vi "example test.vi"() -> ()   [LabVIEW 2013, in "scan engine tests.lvlib"]
uses:
  scan engine tests.lvlib
  <vilib>/NI/Tag Bus/table/allocation specification.ctl
  <vilib>/NI/Tag Bus/tag/Data Type.ctl
  <vilib>/NI/Tag Bus/dictionary/full data dictionary.ctl
  configuration/Scan Engine configuration.lvclass
  execution/Scan Engine runtime.lvclass
  <vilib>/NI/Tag Bus Module Framework/channel/channel classification.ctl
  configuration/Scan Engine configuration.lvclass/Scan Engine configuration.ctl
  <vilib>/NI/Tag Bus/table/data polymorphs/write one/write Boolean.vi
  <vilib>/NI/Tag Bus/table/data polymorphs/read one/read Double.vi
  configuration/Write discover channels.vi
  <vilib>/NI/Tag Bus/table/data table.lvlib
  <vilib>/NI/Tag Bus/dictionary/data dictionary.lvclass
  <vilib>/NI/Tag Bus Module Framework/channel/TBM channel.lvclass
  <vilib>/NI/Tag Bus/tag/tag descriptor.lvclass
panel:
  out "out":T1
  out "in":T1
  in  "do0 value":bool
  out "usec/run out":dbl
  out "usec/run in":dbl
  out "input count":T2[](array[typedef])
  out "output count":T2[](array[typedef])
  in  "for count":i32=1000
  out "AI0 value":dbl
  out "final error":errorcluster
  out "output error":errorcluster
  out "input error":errorcluster
  out "output lookup error":errorcluster
  out "input lookup error":errorcluster
  out "init error":errorcluster
  out "correct execution settings":bool
  out "serialization problem":errorcluster
  out "invalid configuration":errorcluster
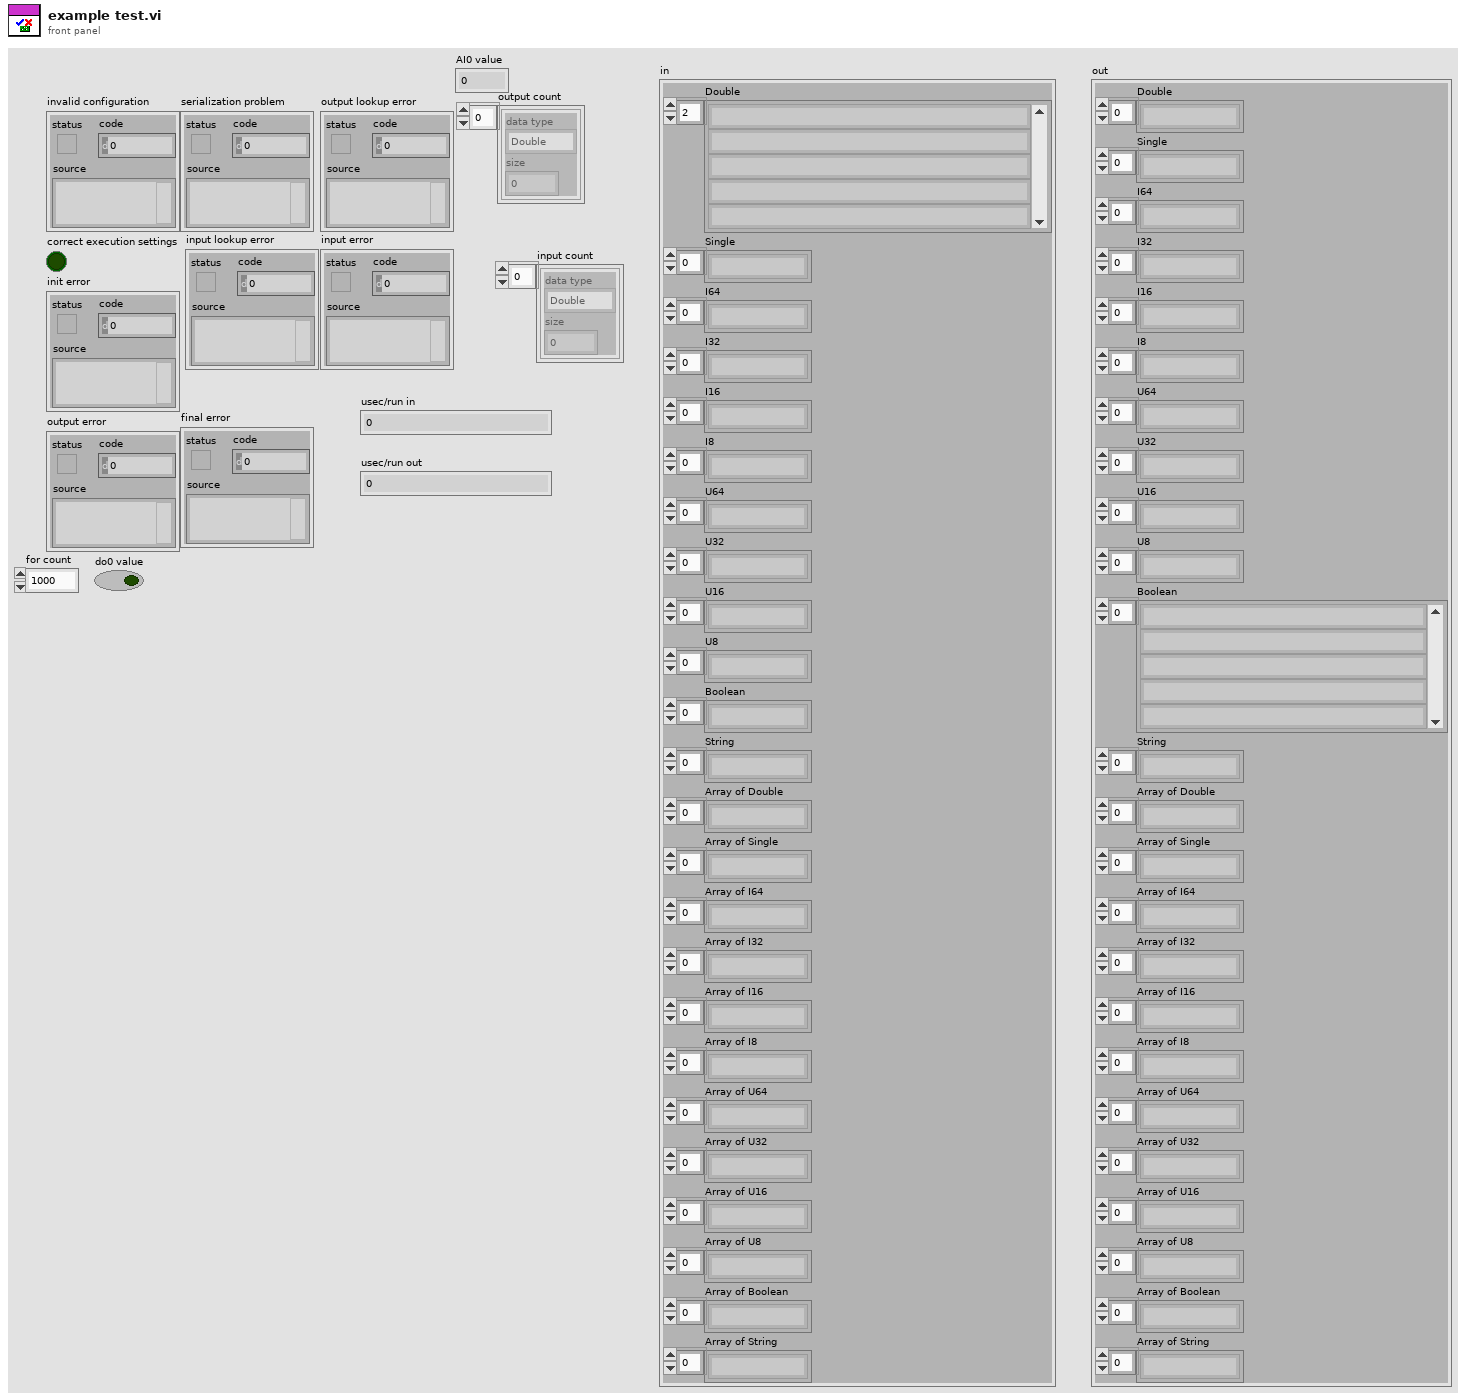
[diagram p1: front panel]
types:
  T1 = typedef "tag bus.lvlib/data dictionary.lvclass/full data dictionary.ctl" = cluster{"Double":string[], "Single":string[], "I64":string[], "I32":string[], "I16":string[], "I8":string[], "U64":string[], "U32":string[], "U16":string[], "U8":string[], "Boolean":string[], "String":string[], "Array of Double":string[], "Array of Single":string[], "Array of I64":string[], "Array of I32":string[], "Array of I16":string[], "Array of I8":string[], "Array of U64":string[], "Array of U32":string[], "Array of U16":string[], "Array of U8":string[], "Array of Boolean":string[], "Array of String":string[]}
  T2 = typedef "tag bus.lvlib/data table.lvlib/allocation specification.ctl" = cluster{"data type":T3, "size":i32}
  T3 = typedef "tag bus.lvlib/tag descriptor.lvclass/Data Type.ctl" = enum16{"Double", "Single", "I64", "I32", "I16", "I8", "U64", "U32", "U16", "U8", "Boolean", "String", "Array of Double", "Array of Single", "Array of I64", "Array of I32", "Array of I16", "Array of I8", "Array of U64", "Array of U32", "Array of U16", "Array of U8", "Array of Boolean", "Array of String"}
  T4 = typedef "TBM channel.lvclass/channel classification.ctl" = enum16{"input data", "output data", "processing parameter", "processing result"}
  T5 = typedef "TBM channel.lvclass/data tables.ctl" = cluster{"input data":T6, "processing parameter":T6, "processing result":T6, "output data":T6}
  T6 = typedef "tag bus.lvlib/dictionary table pair.ctl" = cluster{"data dictionary":refnum<class "data dictionary.lvclass">, "data table":T7}
  T7 = typedef "tag bus.lvlib/data table.lvlib/data table.ctl" = cluster{"Double":dbl[], "Single":sgl[], "I64":i64[], "I32":i32[], "I16":i16[], "I8":i8[], "U64":u64[], "U32":u32[], "U16":u16[], "U8":u8[], "Boolean":bool[], "String":string[], "Array of Double":cluster{"DBL Array":dbl[]}[], "Array of Single":cluster{"SGL Array":sgl[]}[], "Array of I64":cluster{"I64 Array":i64[]}[], "Array of I32":cluster{"I32 Array":i32[]}[], "Array of I16":cluster{"I16 Array":i16[]}[], "Array of I8":cluster{"I8 Array":i8[]}[], "Array of U64":cluster{"U64 Array":u64[]}[], "Array of U32":cluster{"U32 Array":u32[]}[], "Array of U16":cluster{"U16 Array":u16[]}[], "Array of U8":cluster{"U8 Array":u8[]}[], "Array of Boolean":cluster{"Boolean Array":bool[]}[], "Array of String":cluster{"String Array":string[]}[]}
  T8 = typedef "TBM module execution interface.lvclass/execution settings.ctl" = cluster{"reads inputs":bool, "processes data":bool, "writes outputs":bool}
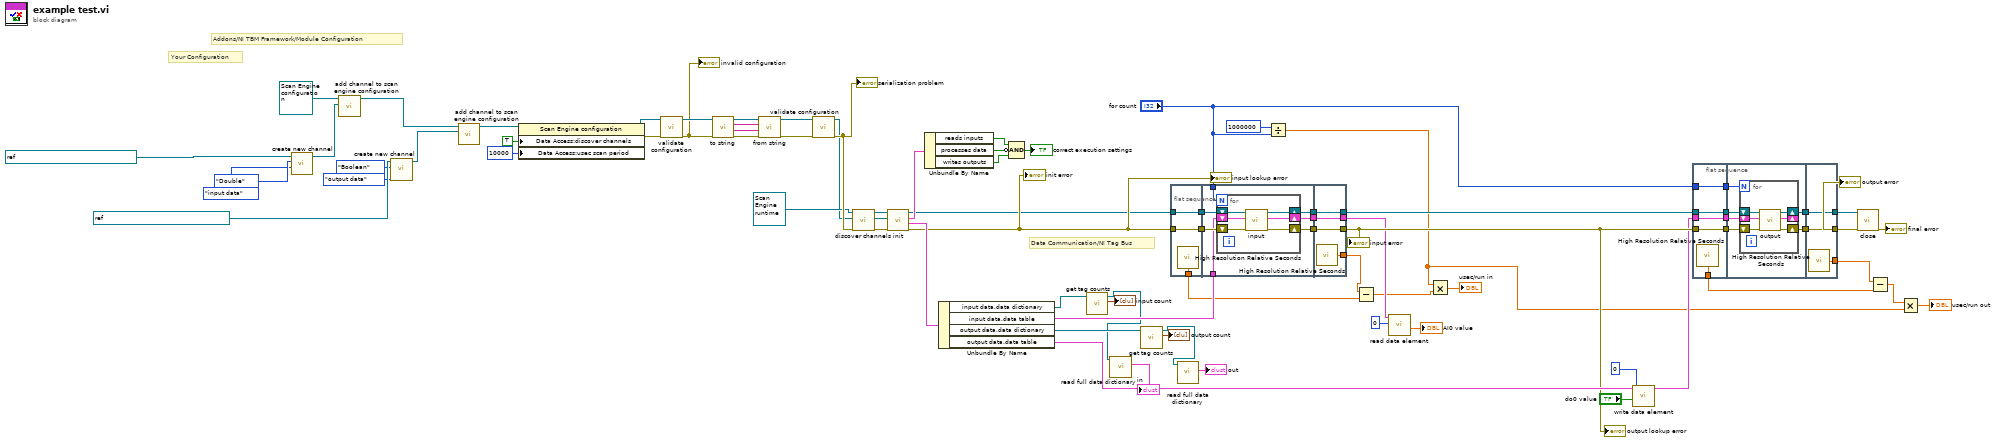
[diagram p0: block diagram]
diagram:
  # "Data Communication/NI Tag Bus"
  # "Your Configuration"
  # "Addons/NI TBM Framework/Module Configuration"
  n1 = call <vilib>:"create new channel.vi"("channel classification"=channel_classification."input data", "data type"=Data_Type."Double", "channel name"=refnum<k21> "ni.var.io://localhost/Mod1/AI0" ("shared variable refnum in")) -> ("channel"=w14:refnum<class "TBM channel.lvclass">)  [unwired: 8 in]
  n2 = call "add channel to scan engine configuration.vi"("channel"=w14, "Scan Engine configuration in"=refnum<class "Scan Engine configuration.lvclass"> refnum ("Scan Engine configuration")) -> ("Scan Engine configuration out"=w15:refnum<class "Scan Engine configuration.lvclass">)  [unwired: 8 in, 1 out]
  n3 = call <vilib>:"create new channel.vi"("channel classification"=channel_classification."output data", "data type"=Data_Type."Boolean", "channel name"=refnum<k21> "ni.var.io://localhost/Mod2/DO0" ("shared variable refnum in")) -> ("channel"=w13:refnum<class "TBM channel.lvclass">)  [unwired: 8 in]
  n4 = call "add channel to scan engine configuration.vi"("channel"=w13, "Scan Engine configuration in"=w15) -> ("Scan Engine configuration out"=w16:refnum<class "Scan Engine configuration.lvclass">)  [unwired: 8 in, 1 out]
  n5 = property class="Scan Engine configuration"(reference=w16, "Data Access:discover channels"=TRUE ("discover channels"), "Data Access:usec scan period"=u32 10000 ("scan period (uSec)")) -> (reference out=w56:refnum<class "Scan Engine configuration.lvclass">, error out=w55:errorcluster)  [unwired: 1 in]
  n6 = call-dynamic "validate configuration.vi"("error in"=w55, "Scan Engine configuration in"=w56) -> ("error out"=w79:errorcluster, "Scan Engine configuration out"=w80:refnum<class "Scan Engine configuration.lvclass">)  [unwired: 8 in]
  "invalid configuration" <- w79
  n7 = call-dynamic "to string.vi"("error in"=w79, "Scan Engine configuration in"=w80) -> ("error out"=w75:errorcluster, "data"=w76:string, "version"=w77:string, "Scan Engine configuration out"=w78:refnum<class "Scan Engine configuration.lvclass">)  [unwired: 6 in]
  n8 = call-dynamic "from string.vi"("error in"=w75, "data"=w76, "version"=w77, "Scan Engine configuration in"=w78) -> ("error out"=w73:errorcluster, "Scan Engine configuration out"=w74:refnum<class "Scan Engine configuration.lvclass">)  [unwired: 6 in]
  n9 = call-dynamic "validate configuration.vi"("error in"=w73, "Scan Engine configuration in"=w74) -> ("error out"=w51:errorcluster, "Scan Engine configuration out"=w46:refnum<class "Scan Engine configuration.lvclass">)  [unwired: 8 in]
  "serialization problem" <- w51
  n10 = call-dynamic "discover channels.vi"("error in"=w51, "module configuration"=w46, "module in"=refnum<class "Scan Engine runtime.lvclass"> refnum ("Scan Engine runtime")) -> ("error out"=w50:errorcluster, "updated configuration"=w49:refnum<class "TBM module configuration.lvclass">, "module out"=w48:refnum<class "Scan Engine runtime.lvclass">)  [unwired: 6 in]
  n11 = call-dynamic "init.vi"("error in"=w50, "TBM module configuration in"=w49, "Scan Engine runtime in"=w48) -> ("error out"=w66:errorcluster, "data allocations"=w67:T5, "execution settings"=w72:T8, "Scan Engine runtime out"=w64:refnum<class "Scan Engine runtime.lvclass">)  [unwired: 5 in]
  "init error" <- w66
  "input lookup error" <- w66
  n12 = Unbundle By Name(w72) -> ("reads inputs"=w69:bool, "processes data"=w71:bool, "writes outputs"=w70:bool)
  n13 = Unbundle By Name(w67) -> ("input data.data dictionary"=w5:refnum<class "data dictionary.lvclass">, "input data.data table"=w65:T7, "output data.data dictionary"=w24:refnum<class "data dictionary.lvclass">, "output data.data table"=w63:T7)
  n14 = Compound Arithmetic op=AND(w69, invert w71, w70) -> (→"correct execution settings":bool)
  n15 = call <vilib>:"get tag counts.vi"("data dictionary in"=w5) -> ("counts"=→"input count":T2[], "data dictionary out"=w1:refnum<class "data dictionary.lvclass">)  [unwired: 9 in]
  n16 = call <vilib>:"read full data dictionary.vi"("data dictionary in"=w1) -> ("dictionary"=→"in":T1)  [unwired: 8 in, 2 out]
  n17 = call <vilib>:"get tag counts.vi"("data dictionary in"=w24) -> ("counts"=→"output count":T2[], "data dictionary out"=w3:refnum<class "data dictionary.lvclass">)  [unwired: 9 in]
  n18 = flat-sequence {
    tunnel: w64 -> [w82]
    tunnel: w66 -> [w83]
    tunnel: [w83] -> w36
    tunnel: [w82] -> w35
    tunnel: [w81] -> w26
    tunnel: w65 -> [w89]
    tunnel: "for count" -> [w84]
    tunnel: w36 -> [w90]
    tunnel: w35 -> [w88]
    tunnel: [w87] -> w34
    tunnel: [w86] -> w33
    tunnel: [w85] -> w32
    tunnel: [w98] -> w45
    tunnel: [w99] -> w61
    tunnel: [w100] -> w62
    tunnel: w34 -> [w100]
    tunnel: w33 -> [w99]
    tunnel: w32 -> [w98]
    tunnel: [w97] -> w27
    frame #0 {
      n19 = call <vilib>:"High Resolution Relative Seconds.vi"() -> ("relative seconds"=w81:dbl)
    }
    frame #1 {
      n20 = for {
        N: w84 -> [_]
        shift-right: [w92] -> w86
        shift-left: w88 -> [w94]
        shift-right: [w93] -> w87
        shift-left: w90 -> [w96]
        shift-right: [w91] -> w85
        shift-left: w89 -> [w95]
        n21 = call-dynamic "input.vi"("error in"=w96, "data table in"=w95, "Scan Engine runtime in"=w94) -> ("error out"=w93:errorcluster, "data table out"=w91:T7, "Scan Engine runtime out"=w92:refnum<class "Scan Engine runtime.lvclass">)  [unwired: 6 in]
      }
    }
    frame #2 {
      n22 = call <vilib>:"High Resolution Relative Seconds.vi"() -> ("relative seconds"=w97:dbl)
    }
  }
  n23 = call <vilib>:"read full data dictionary.vi"("data dictionary in"=w3) -> ("dictionary"=→"out":T1)  [unwired: 8 in, 2 out]
  n24 = Divide(x=1000000, y="for count") -> (x/y=w19:dbl)
  n25 = Subtract(x=w27, y=w26) -> (x-y=w21:dbl)
  n26 = call-poly <vilib>:"read data element.vi"("index"=0, "data table in"=w45) -> ("value"=→"AI0 value":dbl)  [unwired: 8 in, 1 out]
  n27 = Multiply(x=w19, y=w21) -> (x*y=→"usec/run in":dbl)
  n28 = call-poly <vilib>:"write data element.vi"("value"="do0 value", "index"=0, "data table in"=w63) -> ("data table out"=w60:T7)  [unwired: 8 in]
  n29 = flat-sequence {
    tunnel: "for count" -> [w102]
    tunnel: w60 -> [w103]
    tunnel: w61 -> [w104]
    tunnel: w62 -> [w105]
    tunnel: [w105] -> w42
    tunnel: [w104] -> w41
    tunnel: [w103] -> w40
    tunnel: [w102] -> w39
    tunnel: [w101] -> w28
    tunnel: w42 -> [w111]
    tunnel: w41 -> [w110]
    tunnel: w40 -> [w109]
    tunnel: w39 -> [w106]
    tunnel: [w108] -> w38
    tunnel: [w107] -> w37
    tunnel: [w119] -> w58
    tunnel: [w120] -> w59
    tunnel: w38 -> [w120]
    tunnel: w37 -> [w119]
    tunnel: [w118] -> w29
    frame #0 {
      n30 = call <vilib>:"High Resolution Relative Seconds.vi"() -> ("relative seconds"=w101:dbl)
    }
    frame #1 {
      n31 = for {
        N: w106 -> [_]
        shift-right: [w112] -> _
        shift-left: w109 -> [w115]
        shift-right: [w114] -> w108
        shift-left: w110 -> [w116]
        shift-right: [w113] -> w107
        shift-left: w111 -> [w117]
        n32 = call-dynamic "output.vi"("error in"=w117, "data table in"=w115, "Scan Engine runtime in"=w116) -> ("error out"=w113:errorcluster, "data table out"=w112:T7, "Scan Engine runtime out"=w114:refnum<class "Scan Engine runtime.lvclass">)  [unwired: 6 in]
      }
    }
    frame #2 {
      n33 = call <vilib>:"High Resolution Relative Seconds.vi"() -> ("relative seconds"=w118:dbl)
    }
  }
  n34 = call-dynamic "close.vi"("error in"=w58, "Scan Engine runtime in"=w59) -> ("error out"=→"final error":errorcluster)  [unwired: 9 in]
  n35 = Subtract(x=w29, y=w28) -> (x-y=w20:dbl)
  n36 = Multiply(x=w20, y=w19) -> (x*y=→"usec/run out":dbl)
  "output lookup error" <- w62
  "input error" <- w62
  "output error" <- w58
